vi "Agilent SNA Read Trigger Mode (SWP).vi"(6 "Channel":i8=1 min=1 max=99 step=1, 7 "Agilent SNA":T1, 8 "error in (no error)":errorcluster, 11 "VISA Resource Names":T3) -> (0 "error out":errorcluster, 2 "Trigger Mode":T2, 3 "dup VISA Resource Names":T3)   [LabVIEW 2011]
doc: "This VI for the HP8753B Network Analyzers reads the stimulus values. Except when performing log sweeps and freq list sweeps, this VI uses the start and stop values and the number of points to calcuate the stimulus values."
uses:
  TypeDefs/Agilent SNA Trigger Mode.ctl
  TypeDefs/Agilent SNA Instrument Info.ctl
  TypeDefs/Agilent SNA VISA.ctl
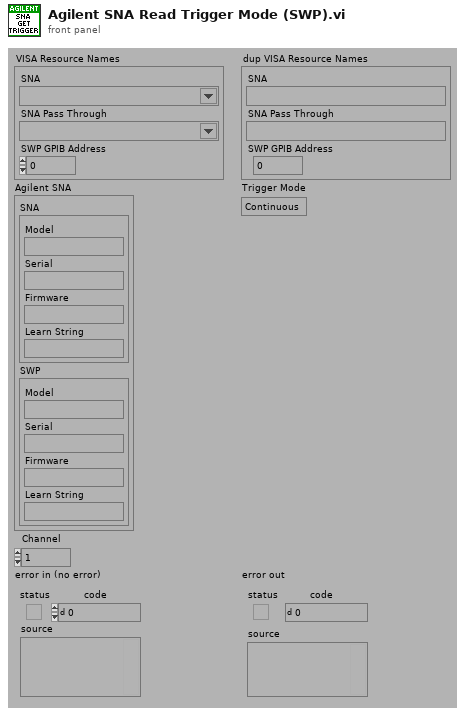
[diagram p1: front panel]
types:
  T1 = typedef "Agilent SNA Instrument Info.ctl" = cluster{"SNA":cluster{"Model":string, "Serial":string, "Firmware":string, "Learn String":string}, "SWP":cluster{"Model":string, "Serial":string, "Firmware":string, "Learn String":string}}
  T2 = typedef "Agilent SNA Trigger Mode.ctl" = enum16{"Continuous", "Hold", "Single"}
  T3 = typedef "Agilent SNA VISA.ctl" = cluster{"SNA":refnum<visa-resource-name>, "SNA Pass Through":refnum<visa-resource-name>, "SWP GPIB Address":i32}
  T4 = typedef "Agilent SNA Model.ctl" = enum16{"Not Supported", "8757X"}
  T5 = typedef "Agilent SNA SWP Model.ctl" = enum16{"Not Supported", "836XXX", "8375XX", "E82X7D"}
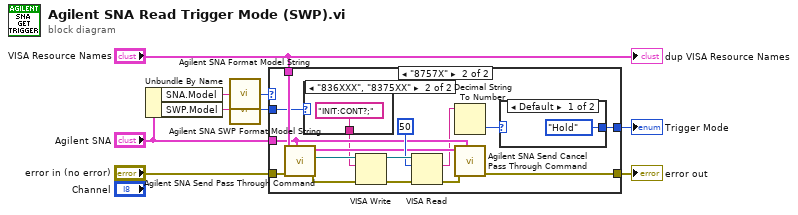
[diagram p0: block diagram]
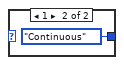
[diagram p3: hidden frame]
diagram:
  n1 = Unbundle By Name("Agilent SNA") -> ("SNA.Model"=w9:string, "SWP.Model"=w7:string)
  n2 = call "Agilent SNA Format Model String.vi"("Model String"=w9) -> ("Model"=w8:T4)
  n3 = call "Agilent SNA SWP Format Model String.vi"("Model String"=w7) -> ("Model"=w6:T5)
  n4 = case shown="\"8757X\"" w8 {
    tunnel: "error in (no error)" -> [w10 w23]
    tunnel: [w10 w18] -> w4
    tunnel: [_ w11] -> w1
    tunnel: "Agilent SNA" -> [_ w17]
    tunnel: "VISA Resource Names" -> [_ w20]
    tunnel: w6 -> [_ w14]
    frame "Not Supported" {
    }
    frame "8757X" {
      n5 = call "Agilent SNA Send Pass Through Command.vi"("Agilent SNA & SWP"=w17, "error in (no error)"=w23, "VISA Resource Names"=w20) -> ("error out"=w22:errorcluster, "SNA Pass Through"=w21:refnum<visa-resource-name>, "dup VISA Resource Names"=w16:T3)  [unwired: 6 in]
      n6 = case shown="\"836XXX\", \"8375XX\"" w14 {
        tunnel: [_ "INIT:CONT?;"] -> w13
        frame "Not Supported" {
        }
        frame "836XXX", "8375XX" {
        }
      }
      n7 = VISA Write(VISA resource name=w21, write buffer=w13, error in (no error)=w22) -> (VISA resource name out=w26:refnum<visa-resource-name>, error out=w24:errorcluster)  [unwired: 1 out]
      n8 = VISA Read(VISA resource name=w26, byte count=u32 50, error in (no error)=w24) -> (read buffer=w15:string, error out=w19:errorcluster)  [unwired: 2 out]
      n9 = Decimal String To Number(string=w15) -> (number=w12:i32)  [unwired: 2 in, 1 out]
      n10 = call "Agilent SNA Send Cancel Pass Through Command.vi"("Agilent SNA & SWP"=w17, "error in (no error)"=w19, "VISA Resource Names"=w16) -> ("error out"=w18:errorcluster)  [unwired: 7 in, 1 out]
      n11 = case shown="Default" w12 {
        tunnel: [Agilent_SNA_Trigger_Mode."Hold" Agilent_SNA_Trigger_Mode."Continuous"] -> w11
        frame Default {
        }
        frame 1 {
        }
      }
    }
  }
  "error out" <- w4
  "Trigger Mode" <- w1
  "dup VISA Resource Names" <- "VISA Resource Names"
